vi "Get MeasData from Q.vi"(8 "error in (no error)":errorcluster) -> (0 "error out":errorcluster, 2 "MeasData out":T1, 3 "orData out":T2)   [LabVIEW 2017]
doc: "Developed by Kevin Thompson\nThompson Engineering, LLC\nkevin@thompsonengineering.net"
uses:
  TD MeasData QRef.ctl
  TD MeasData--cluster.ctl
  GBL DataQ Ref.vi
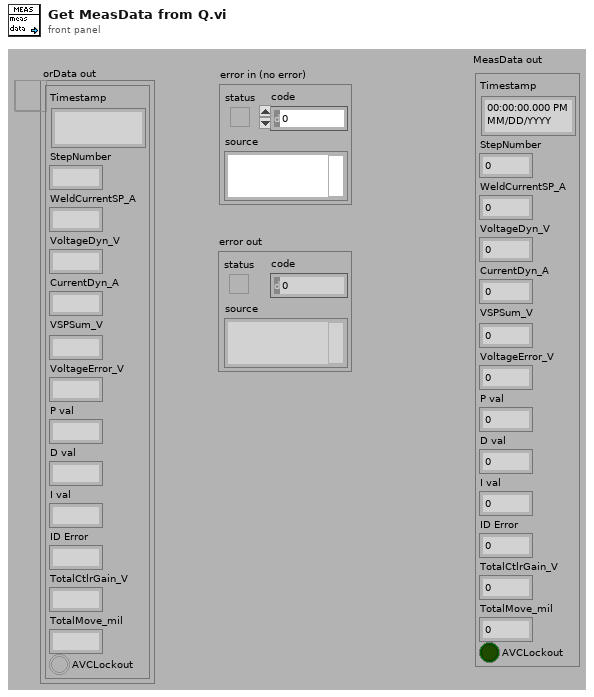
[diagram p1: front panel]
types:
  T1 = typedef "TD MeasData--cluster.ctl" = cluster{"Timestamp":timestamp, "StepNumber":i32, "WeldCurrentSP_A":dbl, "VoltageDyn_V":dbl, "CurrentDyn_A":dbl, "VSPSum_V":dbl, "VoltageError_V":dbl, "P val":dbl, "D val":dbl, "I val":dbl, "ID Error":dbl, "TotalCtlrGain_V":dbl, "TotalMove_mil":dbl, "AVCLockout":bool}
  T2 = typedef "TD MeasData QRef.ctl" = refnum<queue>
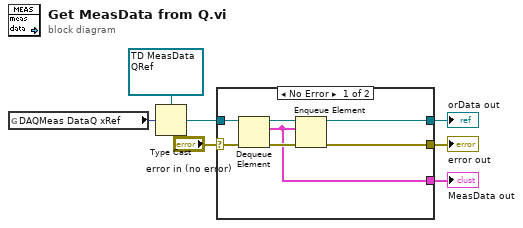
[diagram p0: block diagram]
diagram:
  n1 = global read "GBL DataQ Ref.vi" "DAQMeas DataQ xRef"() -> (w1:u32)
  n2 = Type Cast(type=T2 refnum ("orData in"), x=w1) -> (*(type *) &x=w3:T2)
  n3 = case shown="No Error" "error in (no error)" {
    selector: "error in (no error)" -> [w9 w15]
    tunnel: w3 -> [w14 w16]
    tunnel: [w11 w15] -> w7
    tunnel: [w10 w16] -> w6
    tunnel: [w8 _] -> w2
    frame No Error {
      n4 = Dequeue Element(queue=w14, error in (no error)=w9) -> (queue out=w12:T2, element=w8:T1, error out=w13:errorcluster)  [unwired: 1 in, 1 out]
      n5 = Enqueue Element(queue=w12, element=w8, error in (no error)=w13) -> (queue out=w10:T2, error out=w11:errorcluster)  [unwired: 1 in, 1 out]
    }
    frame Error {
    }
  }
  "orData out" <- w6
  "error out" <- w7
  "MeasData out" <- w2
